vi "Feed Module Tags.vi"(0 "Feed Module Configs":T1[](array[typedef]) {"Settings"."output range"."output low" min=0.0 max=100.0 format="%.2f"; "Settings"."output range"."output high" format="%.2f"; "Settings"."PID 2 Parameters"."PID gains"."derivative time (Td, min)" format="%.3f"; "Settings"."PID 2 Parameters"."PID gains"."integral time (Ti, min)" format="%.3f"; "Settings"."PID 2 Parameters"."PID gains"."proportional gain (Kc)" format="%.3f"; "Settings"."ASIA Pump C"."channel" min=0 max=1 step=1; "Settings"."Ismatech"."Pump Number" min=1.0 max=20.0 step=1.0; "Settings"."Masterflex"."Pump Number" min=1.0 max=20.0 step=1.0}) -> (2 "All  Flow Meter Tags":string[](array[string]), 3 "All  Scale Tags":string[](array[string]), 4 "All  Numeric Tags":string[](array[string]), 6 "Pump Flow Tag":string, 8 "Feed Module Tag Names":T18, 10 "Feed Module Tags Array":T18[](array[typedef]), 12 "Scale Tag":string, 13 "All Boolean Tags":string[](array[string]), 14 "PID 2 Out Tag":string)   [LabVIEW 2018]
uses:
  Feed Module/Controls/Feed Module Tag Names Cluster.ctl
  Feed Module/Controls/Feed Module Config Cluster.ctl
  <vilib>/Utility/miscctls.llb/LVPoint32TypeDef.ctl
  Feed Module/Controls/Feed Module Settings Cluster.ctl
  Ismatec ISM 831C/Controls/Ismatech Settings Cluster.ctl
  Masterflex 7550-30/Controls/Settings Cluster.ctl
  Mettler Toledo/Controls/Settings Cluster.ctl
  Bronkhorst M13 Flow Meter/Settings Cluster.ctl
  Measure Instrument/PID 2 Parameters Cluster.ctl
  Measure Instrument/PID Input Enum.ctl
  Measure Instrument/PID 2 Output Enum.ctl
  Tacmina QI/Tacmina QI DAQ Setting.ctl
  KNF Pump/Settings Cluster plus SIMDOS.ctl
  ASIA Pump/Pump Settings.ctl
  VICI M50 Party Mode/Settings Cluster.ctl
  FLOM Pump/Settings Cluster.ctl
  SSI PR Class/SSI PR or LD Settings Cluster.ctl
  Masterflex 75211/Masterflex 75211 DAQ Setting.ctl
  Feed Module/Feed Module.lvlib
  Masterflex 7550-30/Masterflex 7550-30.lvlib
  Ismatec ISM 831C/Ismatec ISM 831C.lvlib
  Tacmina QI/Tacmina QI.lvlib
  KNF Pump/KNF SIMDOS.lvlib
  VICI M50 Party Mode/VICI M6 M50 Party Mode.lvlib
  FLOM Pump/FLOM Pump.lvlib
  ASIA Pump.lvlib
  Mettler Toledo/Mettler Toledo.lvlib
  Bronkhorst M13 Flow Meter/Bronkhorst M13 Flow Meter.lvlib
  SSI PR Class/SSI PR or LD Pump.lvlib
  Masterflex 75211/Masterflex 75211.lvlib
panel:
  # "Output Instruments"
  # "Input Instruments"
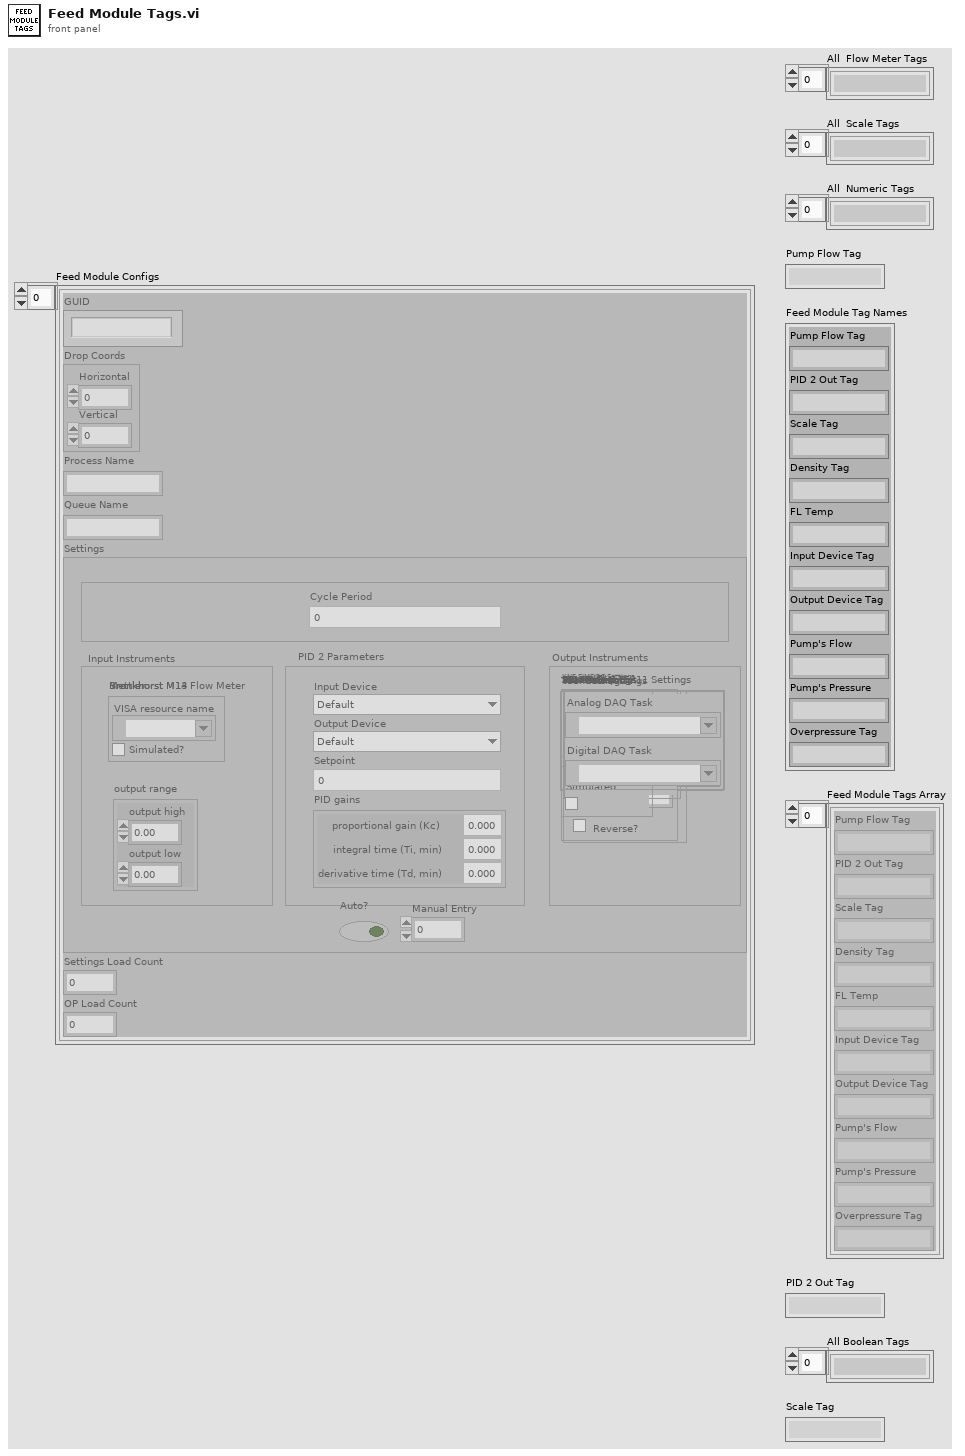
[diagram p1: front panel]
types:
  T1 = typedef "Feed Module.lvlib/Feed Module Config Cluster.ctl" = cluster{"GUID":string, "Drop Coords":T2, "Process Name":string, "Queue Name":string, "Settings":T3, "Settings Load Count":i32, "OP Load Count":i32}
  T2 = typedef "LVPoint32TypeDef.ctl" = cluster{"Horizontal":i32, "Vertical":i32}
  T3 = typedef "Feed Module.lvlib/Feed Module Settings Cluster.ctl" = cluster{"Cycle Period":dbl, "Ismatech":T4, "Masterflex":T5, "Mettler":T6, "Bronkhorst M13 Flow Meter":T7, "PID 2 Parameters":T8, "Manual Entry":dbl, "Auto?":bool, "output range":cluster{"output high":dbl, "output low":dbl}, "Bronkhorst M14":T6, "Tacmina Settings":T11, "KNF SIMDOS Settings":T12, "ASIA Pump C":T13, "VICI Settings":T14, "FLOM Settings":T15, "SSI PR Settings":T16, "Masterflex 75211 Settings":T17}
  T4 = typedef "Ismatec ISM 831C.lvlib/Ismatech Settings Cluster.ctl" = cluster{"VISA resource name":refnum<visa-resource-name>, "Simulated?":bool, "Pump Number":dbl, "Reverse?":bool}
  T5 = typedef "Masterflex 7550-30.lvlib/Settings Cluster.ctl" = cluster{"VISA resource name":refnum<visa-resource-name>, "Simulated?":bool, "Pump Number":dbl, "Reverse?":bool}
  T6 = typedef "Mettler Toledo.lvlib/Settings Cluster.ctl" = cluster{"VISA resource name":refnum<visa-resource-name>, "Simulated?":bool}
  T7 = typedef "Bronkhorst M13 Flow Meter.lvlib/Settings Cluster.ctl" = cluster{"VISA resource name":refnum<visa-resource-name>, "Simulated?":bool}
  T8 = typedef "PID 2 Parameters Cluster.ctl" = cluster{"Input Device":T9, "Output Device":T10, "Setpoint":dbl, "PID gains":cluster{"proportional gain (Kc)":dbl, "integral time (Ti, min)":dbl, "derivative time (Td, min)":dbl}}
  T9 = typedef "PID Input Enum.ctl" = enum16{"Default", "Bronkhorst M13", "Bronkhorst M14", "Scale Rate of Change"}
  T10 = typedef "PID 2 Output Enum.ctl" = enum16{"Default", "Ismatec ISM 831C", "Masterflex 7550-30", "VICI", "Tacmina QI", "KNF SIMDOS", "ASIA Type C", "FLOM UI-22-11", "SSI PR", "Masterflex 75211-70"}
  T11 = typedef "Tacmina QI.lvlib/Tacmina QI DAQ Setting.ctl" = cluster{"Analog DAQ Task":refnum<k21>, "Digital DAQ Task":refnum<k21>}
  T12 = typedef "KNF SIMDOS.lvlib/Settings Cluster plus SIMDOS.ctl" = cluster{"VISA resource name":refnum<visa-resource-name>, "Simulated?":bool}
  T13 = typedef "ASIA Pump.lvlib/Pump Settings.ctl" = cluster{"ASIA Pump #":i32, "channel":i32, "Simulated":bool}
  T14 = typedef "VICI M6 M50 Party Mode.lvlib/Settings Cluster.ctl" = cluster{"VISA resource name":refnum<visa-resource-name>, "Simulated?":bool, "Pump Letter":string, "Reverse?":bool}
  T15 = typedef "FLOM Pump.lvlib/Settings Cluster.ctl" = cluster{"VISA resource name":refnum<visa-resource-name>, "Simulated?":bool, "Pump Number":dbl}
  T16 = typedef "SSI PR or LD Pump.lvlib/SSI PR or LD Settings Cluster.ctl" = cluster{"VISA resource name":refnum<visa-resource-name>, "Simulated?":bool}
  T17 = typedef "Masterflex 75211.lvlib/Masterflex 75211 DAQ Setting.ctl" = cluster{"Analog DAQ Task":refnum<k21>, "Digital DAQ Task":refnum<k21>}
  T18 = typedef "Feed Module.lvlib/Feed Module Tag Names Cluster.ctl" = cluster{"Pump Flow Tag":string, "PID 2 Out Tag":string, "Scale Tag":string, "Density Tag":string, "FL Temp":string, "Input Device Tag":string, "Output Device Tag":string, "Pump's Flow":string, "Pump's Pressure":string, "Overpressure Tag":string}
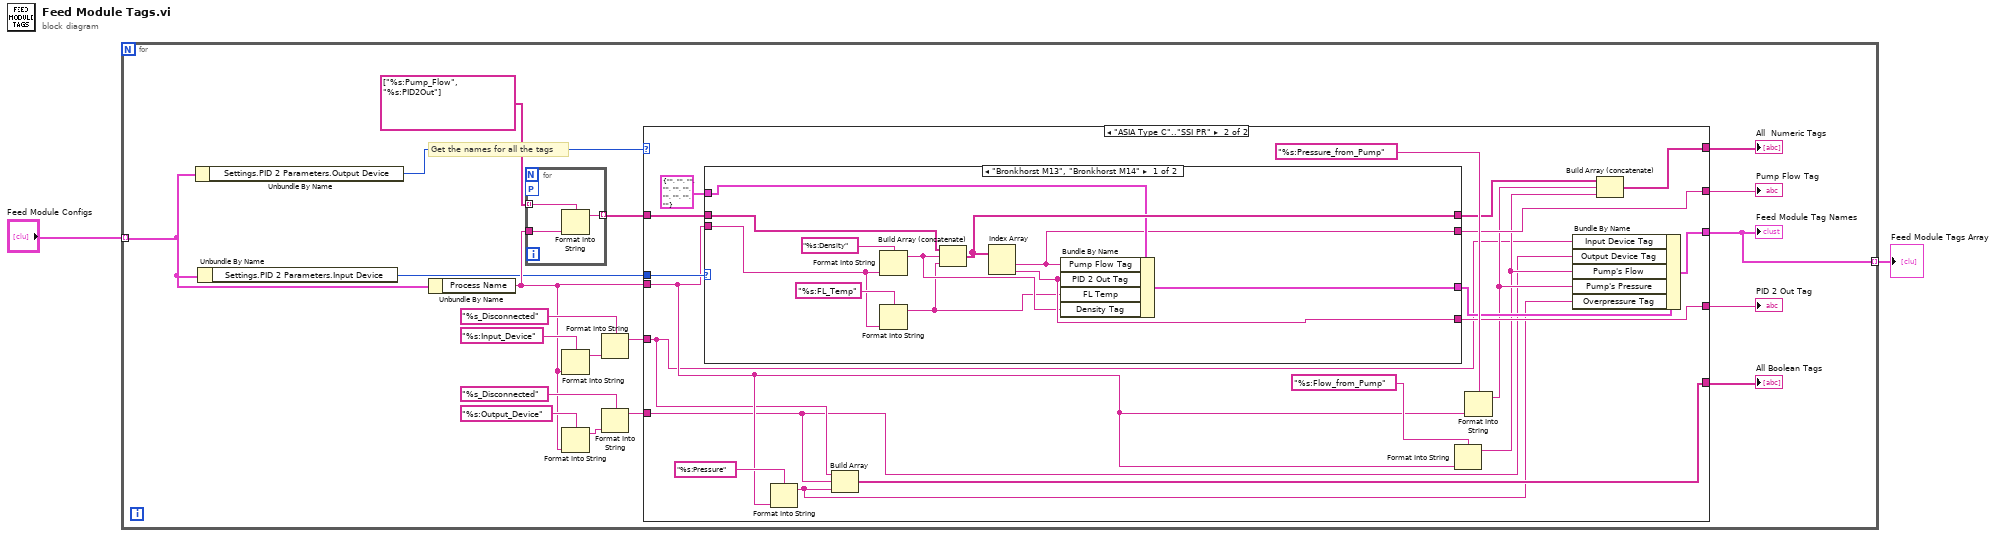
[diagram p0: block diagram]
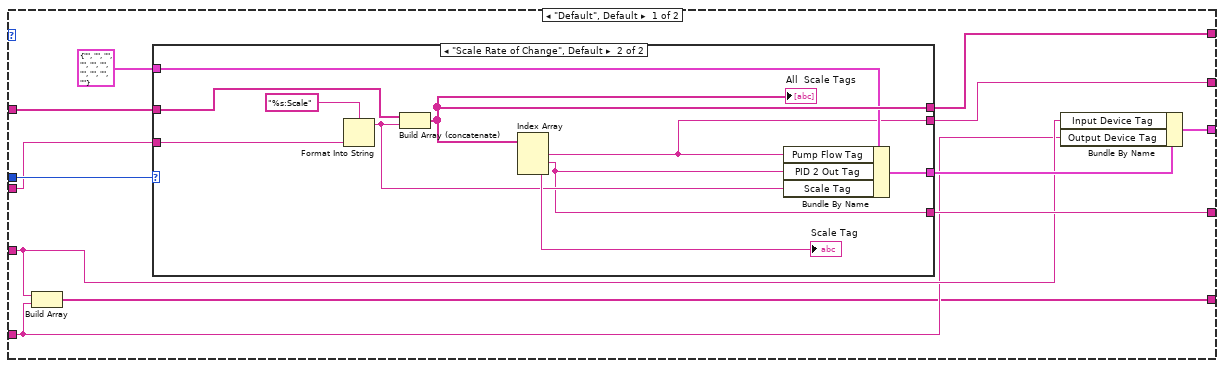
[diagram p2: hidden frame]
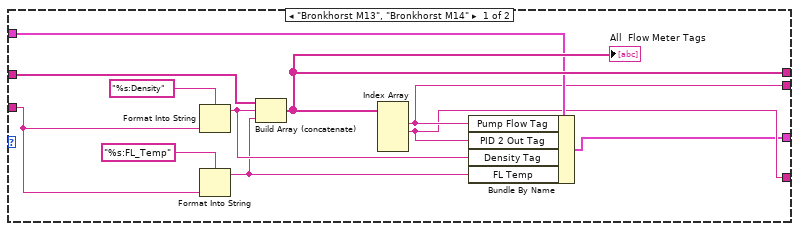
[diagram p3: hidden frame]
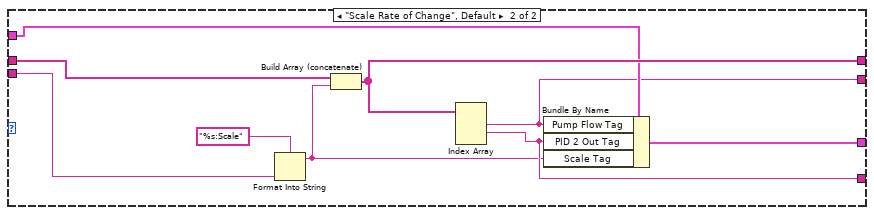
[diagram p4: hidden frame]
diagram:
  n1 = for {
    tunnel: "Feed Module Configs" -> [w4] mode=indexing
    tunnel: [w3] -> w2 mode=indexing
    # "Get the names for all the tags"
    n2 = Unbundle By Name(w4) -> ("Settings.PID 2 Parameters.Output Device"=w14:T10)
    n3 = Unbundle By Name(w4) -> ("Settings.PID 2 Parameters.Input Device"=w12:T9)
    n4 = Unbundle By Name(w4) -> ("Process Name"=w13:string)
    n5 = for {
      tunnel: string[] ["%s:Pump_Flow", "%s:PID2Out"] -> [w96] mode=indexing
      tunnel: w13 -> [w95]
      tunnel: [w94] -> w11 mode=indexing
      workers-P: _ -> [_]
      n6 = Format Into String(format string=w96, w95) -> (resulting string=w94:string)  [unwired: 2 in, 1 out]
    }
    n7 = Format Into String(format string="%s:Input_Device", w13) -> (resulting string=w18:string)  [unwired: 2 in, 1 out]
    n8 = Format Into String(format string="%s:Output_Device", w13) -> (resulting string=w17:string)  [unwired: 2 in, 1 out]
    n9 = Format Into String(format string="%s_Disconnected", w18) -> (resulting string=w7:string)  [unwired: 2 in, 1 out]
    n10 = Format Into String(format string="%s_Disconnected", w17) -> (resulting string=w6:string)  [unwired: 2 in, 1 out]
    n11 = case shown="\"ASIA Type C\"..\"SSI PR\"" w14 {
      tunnel: w13 -> [w31 w59]
      tunnel: w12 -> [w33 w71]
      tunnel: w11 -> [w32 w70]
      tunnel: [w30 w69] -> w10
      tunnel: [w29 w67] -> w8
      tunnel: [w28 w66] -> w9
      tunnel: [w27 w63] -> w3
      tunnel: w7 -> [w24 w58]
      tunnel: w6 -> [w23 w57]
      tunnel: [w22 w56] -> w5
      frame "Default", Default {
        n12 = Build Array(w24, w23) -> (w22:string[])
        n13 = case shown="\"Scale Rate of Change\", Default" w33 {
          tunnel: w32 -> [w42 w54]
          tunnel: [w40 w51] -> w30
          tunnel: w31 -> [w41 w52]
          tunnel: [w38 w47] -> w28
          tunnel: [w37 w45] -> w29
          tunnel: T18 {"Pump Flow Tag"="", "PID 2 Out Tag"="", "Scale Tag"="", "Density Tag"="", "FL Temp"="", "Input Device Tag"="", "Output Device Tag"="", "Pump's Flow"="", "Pump's Pressure"="", "Overpressure Tag"=""} ("Feed Module Tag Names") -> [w39 w49]
          tunnel: [w36 w48] -> w25
          frame "Bronkhorst M13", "Bronkhorst M14" {
            n14 = Format Into String(format string="%s:Density", w41) -> (resulting string=w35:string)  [unwired: 2 in, 1 out]
            n15 = Format Into String(format string="%s:FL_Temp", w41) -> (resulting string=w34:string)  [unwired: 2 in, 1 out]
            n16 = Build Array (concatenate)(w42, w35, w34) -> (w40:string[])
            "All  Flow Meter Tags" <- w40
            n17 = Index Array(array=w40) -> (element #1=w38:string, element #2=w37:string)  [unwired: 4 in, 2 out]
            n18 = Bundle By Name(cluster=w39, "Pump Flow Tag"=w38, "PID 2 Out Tag"=w37, "Density Tag"=w35, "FL Temp"=w34) -> (w36:T18)
          }
          frame "Scale Rate of Change", Default {
            n19 = Format Into String(format string="%s:Scale", w52) -> (resulting string=w46:string)  [unwired: 2 in, 1 out]
            n20 = Build Array (concatenate)(w54, w46) -> (w51:string[])
            "All  Scale Tags" <- w51
            n21 = Index Array(array=w51) -> (element #1=w47:string, element #2=w45:string, element #3=→"Scale Tag":string)  [unwired: 3 in]
            n22 = Bundle By Name(cluster=w49, "Pump Flow Tag"=w47, "PID 2 Out Tag"=w45, "Scale Tag"=w46) -> (w48:T18)
          }
        }
        n23 = Bundle By Name(cluster=w25, "Input Device Tag"=w24, "Output Device Tag"=w23) -> (w27:T18)
      }
      frame "ASIA Type C".."SSI PR" {
        n24 = case shown="\"Bronkhorst M13\", \"Bronkhorst M14\"" w71 {
          tunnel: w70 -> [w82 w93]
          tunnel: [w80 w90] -> w68
          tunnel: w59 -> [w81 w91]
          tunnel: [w78 w86] -> w66
          tunnel: [w77 w87] -> w67
          tunnel: T18 {"Pump Flow Tag"="", "PID 2 Out Tag"="", "Scale Tag"="", "Density Tag"="", "FL Temp"="", "Input Device Tag"="", "Output Device Tag"="", "Pump's Flow"="", "Pump's Pressure"="", "Overpressure Tag"=""} ("Feed Module Tag Names") -> [w79 w89]
          tunnel: [w76 w88] -> w64
          frame "Bronkhorst M13", "Bronkhorst M14" {
            n25 = Format Into String(format string="%s:Density", w81) -> (resulting string=w75:string)  [unwired: 2 in, 1 out]
            n26 = Format Into String(format string="%s:FL_Temp", w81) -> (resulting string=w74:string)  [unwired: 2 in, 1 out]
            n27 = Build Array (concatenate)(w82, w75, w74) -> (w80:string[])
            n28 = Index Array(array=w80) -> (element #1=w78:string, element #2=w77:string)  [unwired: 2 in]
            n29 = Bundle By Name(cluster=w79, "Pump Flow Tag"=w78, "PID 2 Out Tag"=w77, "FL Temp"=w74, "Density Tag"=w75) -> (w76:T18)
          }
          frame "Scale Rate of Change", Default {
            n30 = Format Into String(format string="%s:Scale", w91) -> (resulting string=w85:string)  [unwired: 2 in, 1 out]
            n31 = Build Array (concatenate)(w93, w85) -> (w90:string[])
            n32 = Index Array(array=w90) -> (element #1=w86:string, element #2=w87:string)  [unwired: 3 in, 1 out]
            n33 = Bundle By Name(cluster=w89, "Pump Flow Tag"=w86, "PID 2 Out Tag"=w87, "Scale Tag"=w85) -> (w88:T18)
          }
        }
        n34 = Format Into String(format string="%s:Pressure", w59) -> (resulting string=w55:string)  [unwired: 2 in, 1 out]
        n35 = Build Array(w58, w57, w55) -> (w56:string[])
        n36 = Format Into String(format string="%s:Flow_from_Pump", w59) -> (resulting string=w61:string)  [unwired: 2 in, 1 out]
        n37 = Format Into String(format string="%s:Pressure_from_Pump", w59) -> (resulting string=w62:string)  [unwired: 2 in, 1 out]
        n38 = Bundle By Name(cluster=w64, "Input Device Tag"=w58, "Output Device Tag"=w57, "Pump's Flow"=w61, "Pump's Pressure"=w62, "Overpressure Tag"=w55) -> (w63:T18)
        n39 = Build Array (concatenate)(w68, w62, w61) -> (w69:string[])
      }
    }
    "All  Numeric Tags" <- w10
    "All Boolean Tags" <- w5
    "PID 2 Out Tag" <- w8
    "Pump Flow Tag" <- w9
    "Feed Module Tag Names" <- w3
  }
  "Feed Module Tags Array" <- w2
